vi "Main Window.vi"() -> ()   [LabVIEW 2015]
panel:
  in  "בחירה חופשית":bool caption="Blank Button"
  in  "ממסר השהייה למפוח מפנה גזים 0410-26308":bool caption="Blank Button"
  in  "ממסר דימום מנוע 0410-26294":bool caption="Blank Button"
  in  "0410-24534 15A ממסר":bool caption="Blank Button"
  in  "0410-19646 10Ax4 ממסר":bool caption="Blank Button"
  in  "תיבת נתיכים סימן 4 0414-83040":bool caption="Blank Button"
  in  "תיבת מפעיל ריצוף 1469-98836":bool caption="Blank Button"
  in  "תיבת הזנה כיס צריח 0410-23813":bool caption="Blank Button"
  in  "Help Button":bool
  in  "Stop Button":bool
  out "error IO":errorcluster
  in  "error":errorcluster
  # "צב\"ד לממסרים ונתיכים"
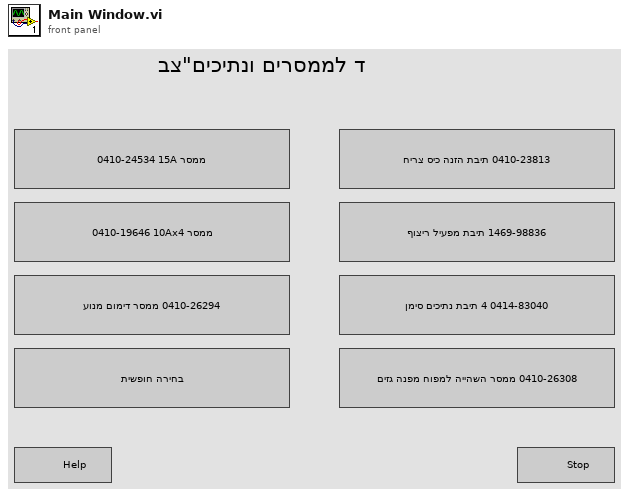
[diagram p1: front panel]
types:
  T1 = enum16{"open", "replace", "create", "open or create", "replace or create", "replace or create with confirmation"}
  T2 = enum32{"Invalid", "Standard", "Closed", "Hidden", "Minimized", "Maximized"}
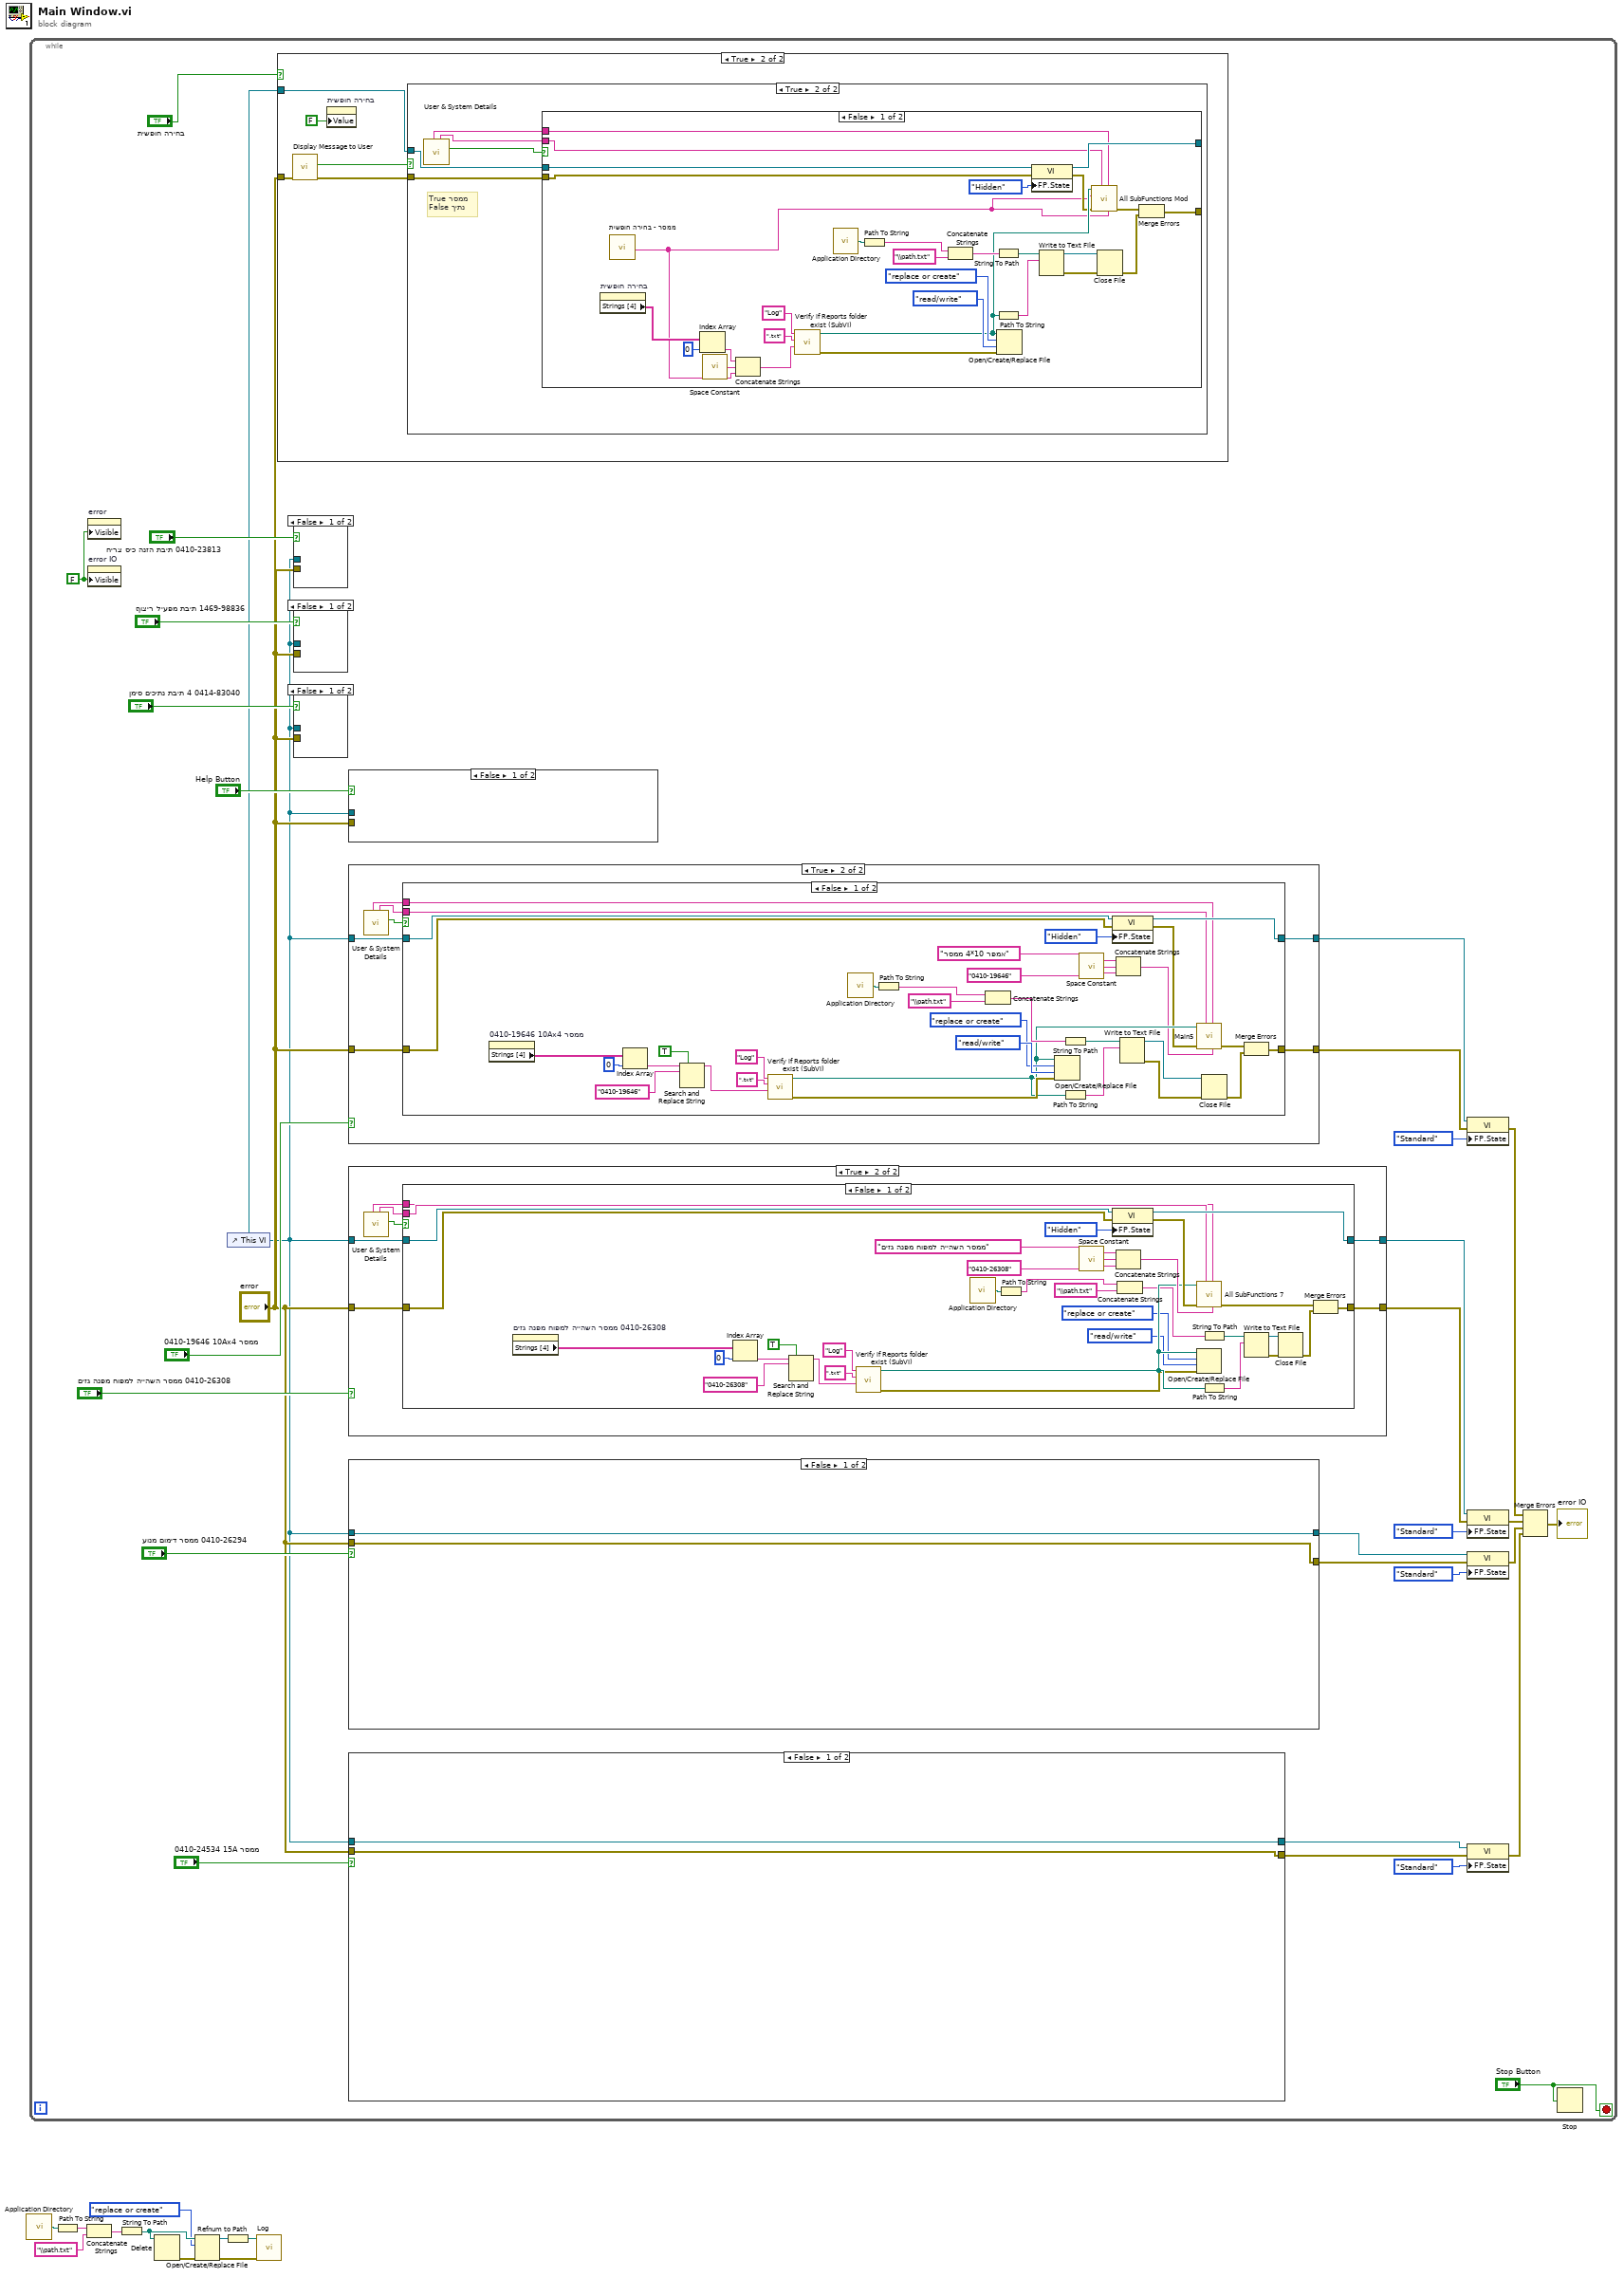
[diagram p0: block diagram]
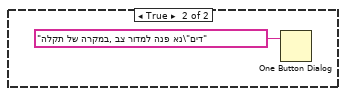
[diagram p5: hidden frame]
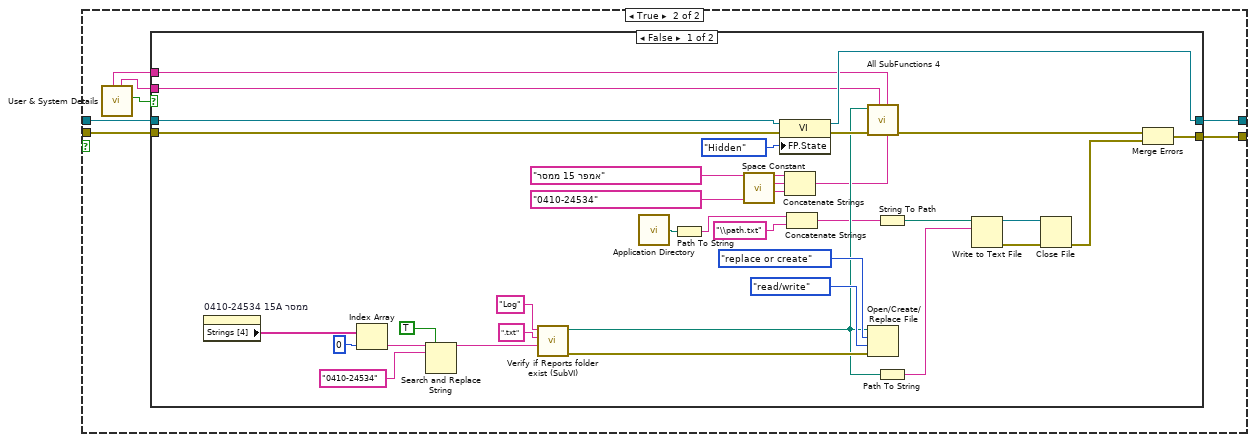
[diagram p6: hidden frame]
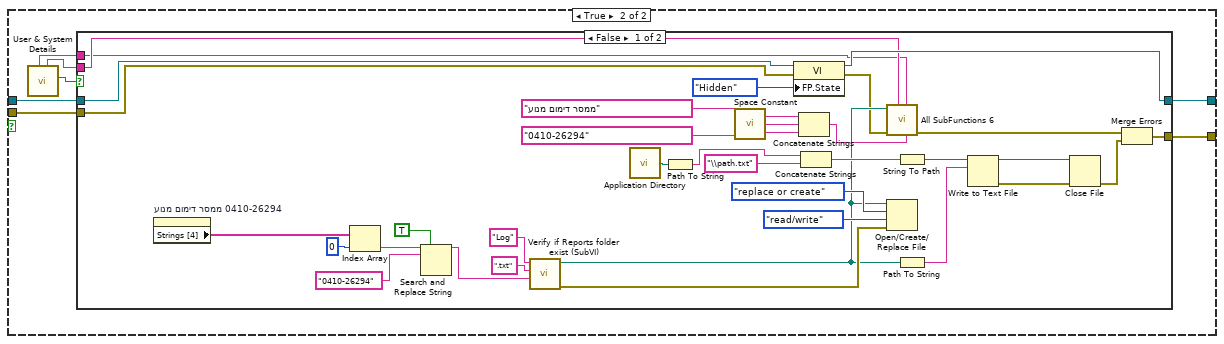
[diagram p13: hidden frame]
diagram:
  n1 = call <vilib>:"Application Directory.vi"() -> ("Application Directory"=w9:path)
  n2 = while {
    stop <- "Stop Button" stop-if-true
    w32 = FALSE ("Visible")
    n3 = property on="error" class="Clust (strict)"("Visible"=w32) -> ()  [unwired: 2 in, 2 out]
    n4 = property on="error IO" class="Clust (strict)"("Visible"=w32) -> ()  [unwired: 2 in, 2 out]
    n5 = control-ref of="This VI"() -> (w12:refnum<vi>)
    n6 = case shown="True" "בחירה חופשית" {
      tunnel: "error" -> [_ w44]
      tunnel: w12 -> [_ w42]
      frame False {
      }
      frame True {
        n7 = call "Display Message to User"("error in (no error)"=w44) -> ("error out"=w43:errorcluster, "ממסר"=w45:bool)  [unwired: 9 in]
        n8 = property on="בחירה חופשית" class="Bool (strict)"("Value"=FALSE ("בחירה חופשית")) -> ()  [unwired: 2 in, 2 out]
        n9 = case shown="True" w45 {
          tunnel: w43 -> [_ w48]
          tunnel: w42 -> [_ w47]
          frame False {
          }
          frame True {
            # "True ממסר\nFalse נתיך"
            n10 = call "User & System Details.vi"() -> ("Boolean"=w46:bool, "User Name 2"=w50:string, "מספר סידורי 2"=w49:string)  [unwired: 9 in]
            n11 = case shown="False" w46 {
              tunnel: w47 -> [w62 w82]
              tunnel: w48 -> [w61 w81]
              tunnel: [w60 w81] -> _
              tunnel: [w59 w82] -> _
              tunnel: w50 -> [w58 _]
              tunnel: w49 -> [w57 _]
              frame False {
                n12 = property on="בחירה חופשית" class="Bool (strict)"() -> ("Strings [4]"=w56:string[])  [unwired: 2 in, 2 out]
                n13 = call "בחירה חופשית - ממסר"() -> ("שם הממסר"=w51:string)  [unwired: 17 in, 2 out]
                n14 = Index Array(array=w56, index=0) -> (element=w54:string)
                n15 = call <vilib>:"Space Constant.vi"() -> ("String"=w53:string)
                n16 = Concatenate Strings(w54, w53, w51) -> (w52:string)
                n17 = call "Verify if Reports folder exist (SubVI).vi"("שם הממסר"=w52, "File Type"=".txt", "Folder Name"="Log" ("string")) -> ("error out"=w69:errorcluster, "Path"=w65:path)  [unwired: 7 in]
                n18 = call <vilib>:"Application Directory.vi"() -> ("Application Directory"=w78:path)
                n19 = Path To String(path=w78) -> (string=w77:string)
                n20 = Concatenate Strings(w77, "\\path.txt") -> (w76:string)
                n21 = String To Path(string=w76) -> (path=w80:path)
                n22 = Path To String(path=w65) -> (string=w72:string)
                n23 = Open/Create/Replace File(file path (use dialog)=w65, error in=w69, operation (0:open)=T1."replace or create", access (0:read/write)=enum16{"read/write", "read-only", "write-only"}."read/write") -> ()  [unwired: 2 in, 3 out]
                n24 = property class="VI"(reference=w62, error in=w61, "FP.State"=T2."Hidden" ("Front Panel Window:State")) -> (reference out=w59:refnum<vi>, error out=w64:errorcluster)
                n25 = Write to Text File(file (use dialog)=w80, text=w72) -> (refnum out=w73:refnum<file>, error out=w74:errorcluster)  [unwired: 2 in, 1 out]
                n26 = call "All SubFunctions Mod.vi"("מק\"ט המכלל"=w51, "מספר סידורי"=w57, "מפעיל"=w58, "error"=w64, "שם הממסר"=w51, "Path for Log"=w65) -> ("error IO"=w63:errorcluster)  [unwired: 5 in]
                n27 = Close File(refnum=w73, error in=w74) -> (error out=w75:errorcluster)  [unwired: 1 out]
                n28 = Merge Errors(w63, w75) -> (w60:errorcluster)
              }
              frame True {
              }
            }
          }
        }
      }
    }
    n29 = case shown="False" "תיבת הזנה כיס צריח 0410-23813" {
      tunnel: w12 -> [_ _]
      tunnel: "error" -> [_ _]
      frame False {
      }
      frame True {
      }
    }
    n30 = case shown="False" "תיבת מפעיל ריצוף 1469-98836" {
      tunnel: w12 -> [_ _]
      tunnel: "error" -> [_ _]
      frame False {
      }
      frame True {
      }
    }
    n31 = case shown="False" "תיבת נתיכים סימן 4 0414-83040" {
      tunnel: "error" -> [_ _]
      tunnel: w12 -> [_ _]
      frame False {
      }
      frame True {
      }
    }
    n32 = case shown="False" "Help Button" {
      tunnel: w12 -> [_ _]
      tunnel: "error" -> [_ _]
      frame False {
      }
      frame True {
        n33 = One Button Dialog(message="במקרה של תקלה, נא פנה למדור צב\"דים") -> ()  [unwired: 1 in, 1 out]
      }
    }
    n34 = case shown="True" "0410-19646 10Ax4 ממסר" {
      tunnel: w12 -> [w129 w137]
      tunnel: "error" -> [w130 w136]
      tunnel: [w130 w135] -> w16
      tunnel: [w129 w134] -> w15
      frame False {
      }
      frame True {
        n35 = call "User & System Details.vi"() -> ("Boolean"=w133:bool, "User Name 2"=w132:string, "מספר סידורי 2"=w131:string)  [unwired: 9 in]
        n36 = case shown="False" w133 {
          tunnel: w137 -> [w143 w173]
          tunnel: w136 -> [w142 w172]
          tunnel: [w141 w172] -> w135
          tunnel: [w140 w173] -> w134
          tunnel: w132 -> [w139 _]
          tunnel: w131 -> [w138 _]
          frame False {
            n37 = property on="0410-19646 10Ax4 ממסר" class="Bool (strict)"() -> ("Strings [4]"=w154:string[])  [unwired: 2 in, 2 out]
            n38 = Index Array(array=w154, index=0) -> (element=w168:string)
            n39 = Search and Replace String(replace all?=TRUE ("replace all? (F)"), input string=w168, search string="0410-19646") -> (result string=w157:string)  [unwired: 5 in, 3 out]
            n40 = call "Verify if Reports folder exist (SubVI).vi"("שם הממסר"=w157, "File Type"=".txt", "Folder Name"="Log" ("string")) -> ("error out"=w151:errorcluster, "Path"=w147:path)  [unwired: 7 in]
            n41 = call <vilib>:"Application Directory.vi"() -> ("Application Directory"=w165:path)
            n42 = Path To String(path=w165) -> (string=w164:string)
            n43 = Concatenate Strings(w164, "\\path.txt") -> (w163:string)
            n44 = Open/Create/Replace File(file path (use dialog)=w147, error in=w151, operation (0:open)=T1."replace or create", access (0:read/write)=enum16{"read/write", "read-only", "write-only"}."read/write") -> ()  [unwired: 2 in, 3 out]
            n45 = String To Path(string=w163) -> (path=w167:path)
            n46 = Path To String(path=w147) -> (string=w159:string)
            n47 = call <vilib>:"Space Constant.vi"() -> ("String"=w169:string)
            n48 = property class="VI"(reference=w143, error in=w142, "FP.State"=T2."Hidden" ("Front Panel Window:State")) -> (reference out=w140:refnum<vi>, error out=w146:errorcluster)
            n49 = Concatenate Strings("ממסר 4*10 אמפר", w169, "0410-19646") -> (w145:string)
            n50 = Write to Text File(file (use dialog)=w167, text=w159) -> (refnum out=w160:refnum<file>, error out=w161:errorcluster)  [unwired: 2 in, 1 out]
            n51 = call "Main5.vi"("מק\"ט המכלל"=w145, "מספר סידורי"=w138, "מפעיל"=w139, "error"=w146, "Path for Log"=w147) -> ("error IO"=w144:errorcluster)  [unwired: 6 in]
            n52 = Close File(refnum=w160, error in=w161) -> (error out=w162:errorcluster)  [unwired: 1 out]
            n53 = Merge Errors(w144, w162) -> (w141:errorcluster)
          }
          frame True {
          }
        }
      }
    }
    n54 = case shown="True" "ממסר השהייה למפוח מפנה גזים 0410-26308" {
      tunnel: "error" -> [w174 w181]
      tunnel: w12 -> [w175 w182]
      tunnel: [w174 w180] -> w20
      tunnel: [w175 w179] -> w19
      frame False {
      }
      frame True {
        n55 = call "User & System Details.vi"() -> ("Boolean"=w178:bool, "User Name 2"=w177:string, "מספר סידורי 2"=w176:string)  [unwired: 9 in]
        n56 = case shown="False" w178 {
          tunnel: w182 -> [w190 w217]
          tunnel: w181 -> [w189 w218]
          tunnel: [w188 w218] -> w180
          tunnel: [w187 w217] -> w179
          tunnel: w177 -> [w184 _]
          tunnel: w176 -> [w183 _]
          frame False {
            n57 = property on="ממסר השהייה למפוח מפנה גזים 0410-26308" class="Bool (strict)"() -> ("Strings [4]"=w206:string[])  [unwired: 2 in, 2 out]
            n58 = Index Array(array=w206, index=0) -> (element=w192:string)
            n59 = Search and Replace String(replace all?=TRUE ("replace all? (F)"), input string=w192, search string="0410-26308") -> (result string=w203:string)  [unwired: 5 in, 3 out]
            n60 = call "Verify if Reports folder exist (SubVI).vi"("שם הממסר"=w203, "File Type"=".txt", "Folder Name"="Log" ("string")) -> ("error out"=w209:errorcluster, "Path"=w213:path)  [unwired: 7 in]
            n61 = call <vilib>:"Application Directory.vi"() -> ("Application Directory"=w195:path)
            n62 = Path To String(path=w195) -> (string=w196:string)
            n63 = call <vilib>:"Space Constant.vi"() -> ("String"=w191:string)
            n64 = property class="VI"(reference=w190, error in=w189, "FP.State"=T2."Hidden" ("Front Panel Window:State")) -> (reference out=w187:refnum<vi>, error out=w214:errorcluster)
            n65 = Concatenate Strings("ממסר השהייה למפוח מפנה גזים", w191, "0410-26308") -> (w215:string)
            n66 = Concatenate Strings(w196, "\\path.txt") -> (w197:string)
            n67 = call "All SubFunctions 7.vi"("מק\"ט המכלל"=w215, "מספר סידורי"=w183, "מפעיל"=w184, "error"=w214, "Path for Log"=w213) -> ("error IO"=w216:errorcluster)  [unwired: 6 in]
            n68 = Open/Create/Replace File(file path (use dialog)=w213, error in=w209, operation (0:open)=T1."replace or create", access (0:read/write)=enum16{"read/write", "read-only", "write-only"}."read/write") -> ()  [unwired: 2 in, 3 out]
            n69 = String To Path(string=w197) -> (path=w193:path)
            n70 = Path To String(path=w213) -> (string=w201:string)
            n71 = Write to Text File(file (use dialog)=w193, text=w201) -> (refnum out=w200:refnum<file>, error out=w199:errorcluster)  [unwired: 2 in, 1 out]
            n72 = Close File(refnum=w200, error in=w199) -> (error out=w198:errorcluster)  [unwired: 1 out]
            n73 = Merge Errors(w216, w198) -> (w188:errorcluster)
          }
          frame True {
          }
        }
      }
    }
    n74 = case shown="False" "ממסר דימום מנוע 0410-26294" {
      tunnel: "error" -> [w219 w227]
      tunnel: w12 -> [w220 w226]
      tunnel: [w220 w225] -> w25
      tunnel: [w219 w224] -> w24
      frame False {
      }
      frame True {
        n75 = call "User & System Details.vi"() -> ("Boolean"=w223:bool, "User Name 2"=w222:string, "מספר סידורי 2"=w221:string)  [unwired: 9 in]
        n76 = case shown="False" w223 {
          tunnel: w227 -> [w237 w263]
          tunnel: w226 -> [w236 w262]
          tunnel: [w235 w262] -> w225
          tunnel: [w234 w263] -> w224
          tunnel: w222 -> [w229 _]
          tunnel: w221 -> [w228 _]
          frame False {
            n77 = property on="ממסר דימום מנוע 0410-26294" class="Bool (strict)"() -> ("Strings [4]"=w244:string[])  [unwired: 2 in, 2 out]
            n78 = Index Array(array=w244, index=0) -> (element=w258:string)
            n79 = Search and Replace String(replace all?=TRUE ("replace all? (F)"), input string=w258, search string="0410-26294") -> (result string=w247:string)  [unwired: 5 in, 3 out]
            n80 = call "Verify if Reports folder exist (SubVI).vi"("שם הממסר"=w247, "File Type"=".txt", "Folder Name"="Log" ("string")) -> ("error out"=w241:errorcluster, "Path"=w233:path)  [unwired: 7 in]
            n81 = call <vilib>:"Application Directory.vi"() -> ("Application Directory"=w255:path)
            n82 = Path To String(path=w255) -> (string=w254:string)
            n83 = call <vilib>:"Space Constant.vi"() -> ("String"=w261:string)
            n84 = property class="VI"(reference=w236, error in=w237, "FP.State"=T2."Hidden" ("Front Panel Window:State")) -> (reference out=w235:refnum<vi>, error out=w232:errorcluster)
            n85 = Concatenate Strings("ממסר דימום מנוע", w261, "0410-26294") -> (w231:string)
            n86 = Concatenate Strings(w254, "\\path.txt") -> (w253:string)
            n87 = call "All SubFunctions 6.vi"("מק\"ט המכלל"=w231, "מספר סידורי"=w228, "מפעיל"=w229, "error"=w232, "Path for Log"=w233) -> ("error IO"=w230:errorcluster)  [unwired: 6 in]
            n88 = Open/Create/Replace File(file path (use dialog)=w233, error in=w241, operation (0:open)=T1."replace or create", access (0:read/write)=enum16{"read/write", "read-only", "write-only"}."read/write") -> ()  [unwired: 2 in, 3 out]
            n89 = String To Path(string=w253) -> (path=w257:path)
            n90 = Path To String(path=w233) -> (string=w249:string)
            n91 = Write to Text File(file (use dialog)=w257, text=w249) -> (refnum out=w250:refnum<file>, error out=w251:errorcluster)  [unwired: 2 in, 1 out]
            n92 = Close File(refnum=w250, error in=w251) -> (error out=w252:errorcluster)  [unwired: 1 out]
            n93 = Merge Errors(w230, w252) -> (w234:errorcluster)
          }
          frame True {
          }
        }
      }
    }
    n94 = case shown="False" "0410-24534 15A ממסר" {
      tunnel: "error" -> [w84 w90]
      tunnel: [w84 w89] -> w30
      tunnel: [w85 w92] -> w28
      tunnel: w12 -> [w85 w91]
      frame False {
      }
      frame True {
        n95 = call "User & System Details.vi"() -> ("Boolean"=w88:bool, "User Name 2"=w87:string, "מספר סידורי 2"=w86:string)  [unwired: 9 in]
        n96 = case shown="False" w88 {
          tunnel: [w125 w127] -> w92
          tunnel: w91 -> [w124 w127]
          tunnel: w90 -> [w112 w128]
          tunnel: [w105 w128] -> w89
          tunnel: w87 -> [w94 _]
          tunnel: w86 -> [w93 _]
          frame False {
            n97 = property on="0410-24534 15A ממסר" class="Bool (strict)"() -> ("Strings [4]"=w117:string[])  [unwired: 2 in, 2 out]
            n98 = Index Array(array=w117, index=0) -> (element=w99:string)
            n99 = Search and Replace String(replace all?=TRUE ("replace all? (F)"), input string=w99, search string="0410-24534") -> (result string=w114:string)  [unwired: 5 in, 3 out]
            n100 = call "Verify if Reports folder exist (SubVI).vi"("שם הממסר"=w114, "File Type"=".txt", "Folder Name"="Log" ("string")) -> ("error out"=w120:errorcluster, "Path"=w111:path)  [unwired: 7 in]
            n101 = call <vilib>:"Application Directory.vi"() -> ("Application Directory"=w102:path)
            n102 = Path To String(path=w102) -> (string=w103:string)
            n103 = call <vilib>:"Space Constant.vi"() -> ("String"=w95:string)
            n104 = property class="VI"(reference=w124, error in=w112, "FP.State"=T2."Hidden" ("Front Panel Window:State")) -> (reference out=w125:refnum<vi>, error out=w123:errorcluster)
            n105 = Concatenate Strings("ממסר 15 אמפר", w95, "0410-24534") -> (w97:string)
            n106 = Concatenate Strings(w103, "\\path.txt") -> (w104:string)
            n107 = call "All SubFunctions 4.vi"("מק\"ט המכלל"=w97, "מספר סידורי"=w93, "מפעיל"=w94, "error"=w123, "Path for Log"=w111) -> ("error IO"=w107:errorcluster)  [unwired: 6 in]
            n108 = Open/Create/Replace File(file path (use dialog)=w111, error in=w120, operation (0:open)=T1."replace or create", access (0:read/write)=enum16{"read/write", "read-only", "write-only"}."read/write") -> ()  [unwired: 2 in, 3 out]
            n109 = String To Path(string=w104) -> (path=w100:path)
            n110 = Path To String(path=w111) -> (string=w110:string)
            n111 = Write to Text File(file (use dialog)=w100, text=w110) -> (refnum out=w109:refnum<file>, error out=w108:errorcluster)  [unwired: 2 in, 1 out]
            n112 = Close File(refnum=w109, error in=w108) -> (error out=w106:errorcluster)  [unwired: 1 out]
            n113 = Merge Errors(w107, w106) -> (w105:errorcluster)
          }
          frame True {
          }
        }
      }
    }
    n114 = property class="VI"(reference=w15, error in=w16, "FP.State"=T2."Standard" ("Front Panel Window:State")) -> (error out=w14:errorcluster)  [unwired: 1 out]
    n115 = property class="VI"(reference=w19, error in=w20, "FP.State"=T2."Standard" ("Front Panel Window:State")) -> (error out=w18:errorcluster)  [unwired: 1 out]
    n116 = property class="VI"(reference=w25, error in=w24, "FP.State"=T2."Standard" ("Front Panel Window:State")) -> (error out=w23:errorcluster)  [unwired: 1 out]
    n117 = property class="VI"(reference=w28, error in=w30, "FP.State"=T2."Standard" ("Front Panel Window:State")) -> (error out=w26:errorcluster)  [unwired: 1 out]
    n118 = Merge Errors(w14, w18, w23, w26) -> (→"error IO":errorcluster)
    n119 = Stop(stop? (T)="Stop Button") -> ()
  }
  n120 = Path To String(path=w9) -> (string=w10:string)
  n121 = Concatenate Strings(w10, "\\path.txt") -> (w7:string)
  n122 = String To Path(string=w7) -> (path=w4:path)
  n123 = Delete(path (use dialog)=w4) -> (error out=w5:errorcluster)  [unwired: 4 in, 2 out]
  n124 = Open/Create/Replace File(file path (use dialog)=w4, error in=w5, operation (0:open)=T1."replace or create") -> (refnum out=w2:refnum<file>, error out=w6:errorcluster)  [unwired: 3 in, 1 out]
  n125 = Refnum to Path(1:w2) -> (0:w1:path)
  n126 = call "Log.vi"("error in"=w6, "File Path Control"=w1) -> ()  [unwired: 8 in, 2 out]
